vi "Z900_navX_Internal_UpdateDevice.vi"(8 "error in (no error)":errorcluster, 10 "Interface TypeDefs":T1 {"I2CDevRef"."Device Address" format="%.0x"}, 11 "navX Device":T7={"Interface"={"Protocol"=enum."SERIAL", "Update Rate (4Hz-60Hz)"=4, "navX Open TypeDef"=variant}, "Notify Packet"=refnum, "Loop VI Refnum"=refnum, "Ready to Close Occurrence Refnum"=refnum} {"Interface"."Update Rate (4Hz-60Hz)" min=4 max=60 step=1}) -> (0 "error out":errorcluster, 2 "Interface TypeDefs":T1 {"I2CDevRef"."Device Address" format="%.0x"}, 3 "navX Device":T7={"Interface"={"Protocol"=enum."SERIAL", "Update Rate (4Hz-60Hz)"=4, "navX Open TypeDef"=variant}, "Notify Packet"=refnum, "Loop VI Refnum"=refnum, "Ready to Close Occurrence Refnum"=refnum} {"Interface"."Update Rate (4Hz-60Hz)" min=4 max=60 step=1})   [LabVIEW 2015, in "navX Library v2.lvlib"]
doc: "This navX VI handles updating rate and serial protocol for the navX.\nTHIS VI SHOULD NOT BE CALLED BY THE USER!"
uses:
  navX Library v2.lvlib
  TypeDefs/Z900_navX_DeviceTypeDef.ctl
  TypeDefs/Z900_navX_ProtocolTypeDef.ctl
  TypeDefs/Z900_navX_NotifyPacketTypeDef.ctl
  TypeDefs/Z900_navX_ActionTypeDef.ctl
  TypeDefs/Z900_navX_InterfaceTypeDef.ctl
  <vilib>/Rock Robotics/WPI/SerialPort/WPI_SerialPortRef.ctl
  <vilib>/Rock Robotics/WPI/I2C/WPI_I2CDevRef.ctl
  <vilib>/Rock Robotics/SystemInterfaces/i2clib/i2c_bus.ctl
  <vilib>/Rock Robotics/WPI/SPI/WPI_SPIDevRef.ctl
  <vilib>/Rock Robotics/SystemInterfaces/spilib/spi_bus.ctl
  TypeDefs/navX Open TypeDefs/Z900_navX_OpenTypeDef_Serial.ctl
  NI WPI/WPI_SerialPort_USB.ctl
  TypeDefs/Z900_navX_SerialStreamTypeDef.ctl
  TypeDefs/navX Open TypeDefs/Z900_navX_OpenTypeDef_I2C.ctl
  TypeDefs/Z900_navX_DeviceRegisters.ctl
  TypeDefs/navX Open TypeDefs/Z900_navX_OpenTypeDef_SPI.ctl
  Desktop/Library Fix Test/NI WPI/NI WPI Serial USB.lvlib
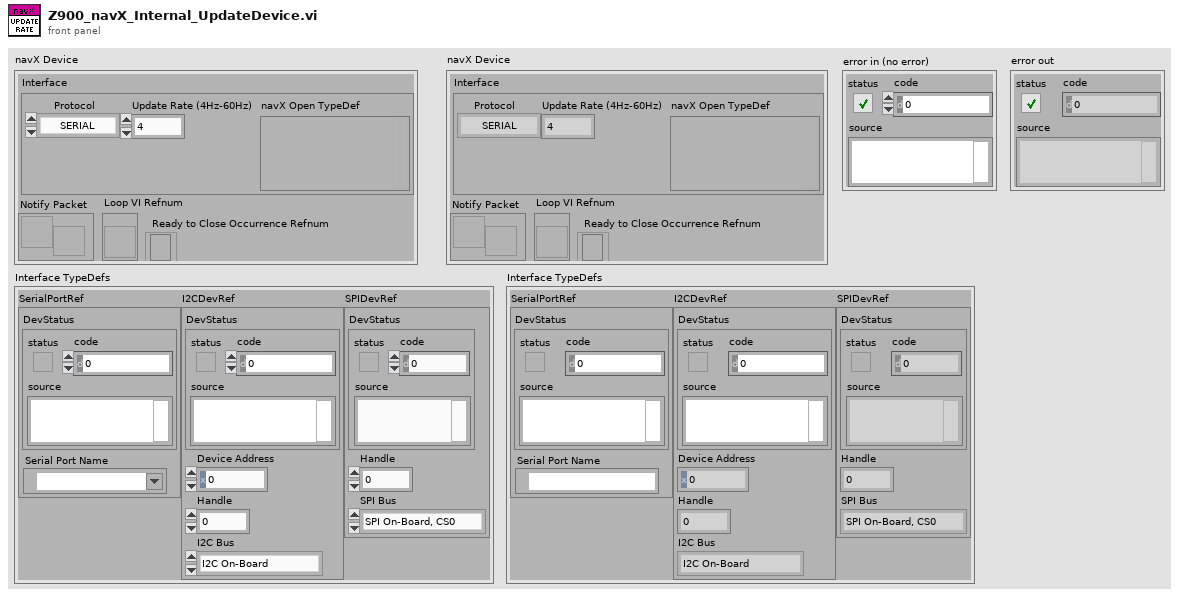
[diagram p1: front panel]
types:
  T1 = typedef "navX Library v2.lvlib/Z900_navX_InterfaceTypeDef.ctl" = cluster{"SerialPortRef":T2, "I2CDevRef":T3, "SPIDevRef":T5}
  T2 = typedef "WPI_SerialPortRef.ctl" = cluster{"DevStatus":errorcluster, "Serial Port Name":refnum<visa-resource-name>}
  T3 = typedef "WPI_I2CDevRef.ctl" = cluster{"DevStatus":errorcluster, "Device Address":u8, "Handle":i32, "I2C Bus":T4}
  T4 = typedef "i2c_bus.ctl" = enum16{"I2C On-Board", "I2C MXP", "Invalid"}
  T5 = typedef "WPI_SPIDevRef.ctl" = cluster{"DevStatus":errorcluster, "Handle":i32, "SPI Bus":T6}
  T6 = typedef "spi_bus.ctl" = enum16{"SPI On-Board, CS0", "SPI On-Board, CS1", "SPI On-Board, CS2", "SPI On-Board, CS3", "SPI MXP", "Invalid"}
  T7 = typedef "navX Library v2.lvlib/Z900_navX_DeviceTypeDef.ctl" = cluster{"Interface":cluster{"Protocol":T8, "Update Rate (4Hz-60Hz)":u8, "navX Open TypeDef":variant}, "Notify Packet":refnum<notifier>, "Loop VI Refnum":refnum<vi>, "Ready to Close Occurrence Refnum":refnum<k4>}
  T8 = typedef "navX Library v2.lvlib/Z900_navX_ProtocolTypeDef.ctl" = enum16{"SERIAL", "I2C", "SPI"}
  T9 = typedef "navX Library v2.lvlib/Z900_navX_OpenTypeDef_Serial.ctl" = cluster{"Serial Port":T10, "Stream Type":T11}
  T10 = typedef "NI WPI Serial USB.lvlib/WPI_SerialPort_USB.ctl" = enum16{"Onboard RS-232", "MXP TTL", "USB"}
  T11 = typedef "navX Library v2.lvlib/Z900_navX_SerialStreamTypeDef.ctl" = enum16{"YRPH", "Quaterinons", "Gyro/Raw", "AHRS", "AHRSAndPositioning"}
  T12 = typedef "navX Library v2.lvlib/Z900_navX_OpenTypeDef_I2C.ctl" = cluster{"I2C Bus":T4}
  T13 = typedef "navX Library v2.lvlib/Z900_navX_OpenTypeDef_SPI.ctl" = cluster{"SPI Bus":T6, "Clock Rate (Hz)":dbl}
  T14 = typedef "navX Library v2.lvlib/Z900_navX_DeviceRegisters.ctl" = u8
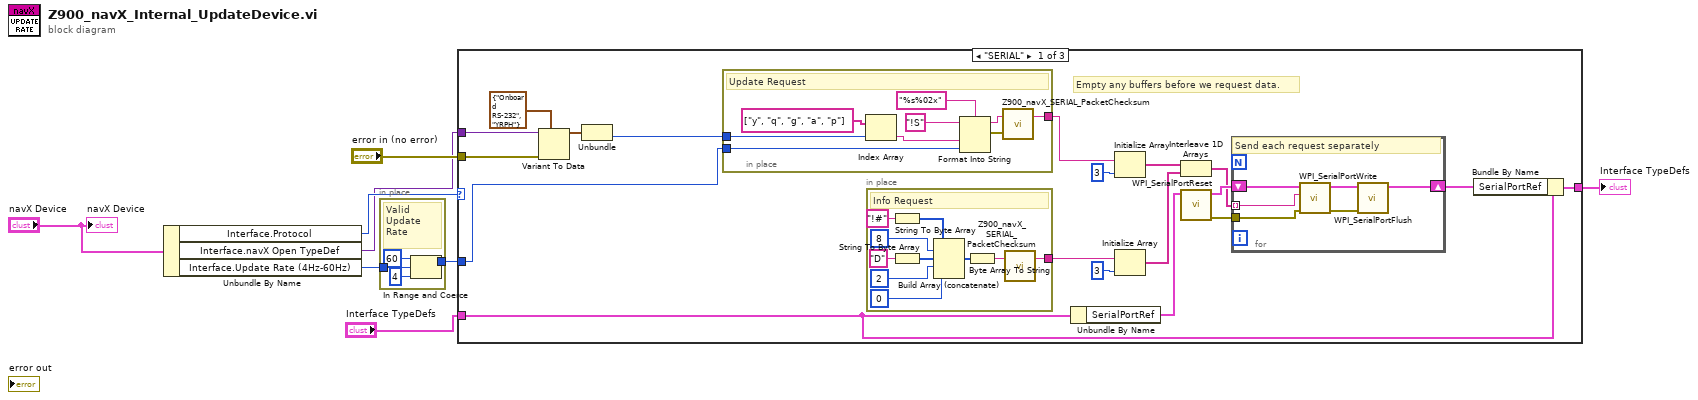
[diagram p0: block diagram]
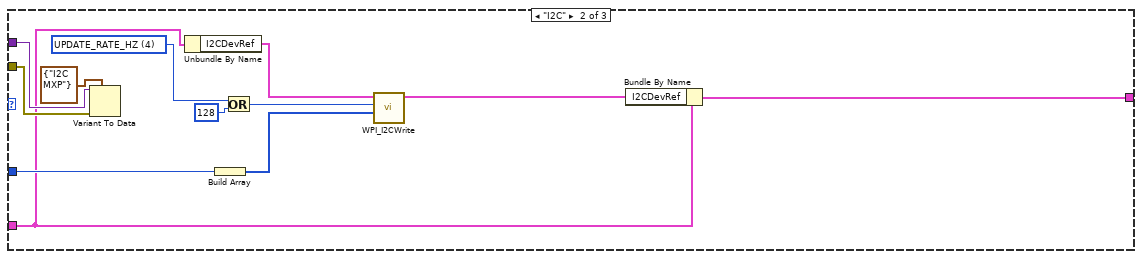
[diagram p2: hidden frame]
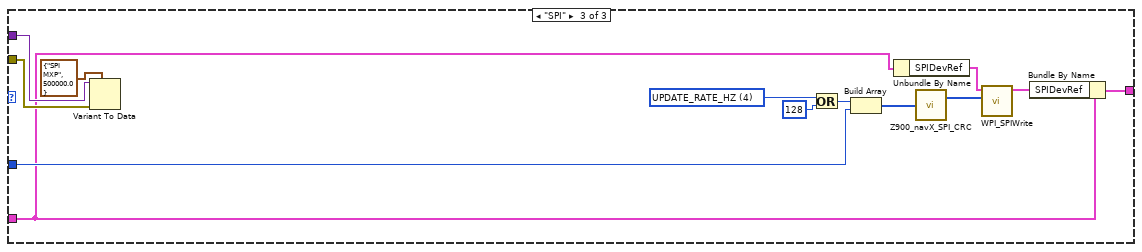
[diagram p3: hidden frame]
diagram:
  n1 = Unbundle By Name("navX Device") -> ("Interface.Protocol"=w7:T8, "Interface.navX Open TypeDef"=w3:variant, "Interface.Update Rate (4Hz-60Hz)"=w2:u8)
  n2 = in-place {
    in-place-border: w2 -> [w12]
    in-place-border: [w9] -> w1
    # "Valid\nUpdate\nRate"
    n3 = In Range and Coerce(upper limit=u8 60, x=w12, lower limit=u8 4) -> (coerced(x)=w9:u8)  [unwired: 1 out]
  }
  n4 = case shown="\"SERIAL\"" w7 {
    tunnel: w3 -> [w31 w68 w81]
    tunnel: "error in (no error)" -> [w29 w66 w79]
    tunnel: "Interface TypeDefs" -> [w26 w59 w71]
    tunnel: w1 -> [w24 w62 w73]
    tunnel: [w25 w57 w69] -> w4
    frame "SERIAL" {
      # "Empty any buffers before we request data."
      n5 = Variant To Data(error in=w29, type=T9 {"Serial Port"=enum."Onboard RS-232", "Stream Type"=enum."YRPH"} ("navX Serial Open"), Variant=w31) -> (data=w28:T9)  [unwired: 1 out]
      n6 = Unbundle(w28) -> ("Stream Type"=w27:T11)  [unwired: 1 out]
      n7 = in-place {
        in-place-border: w27 -> [w45]
        in-place-border: [w38] -> w19
        in-place-border: w24 -> [w39]
        # "Update Request"
        n8 = Index Array(array=string[] ["y", "q", "g", "a", "p"], index=w45) -> (element=w40:string)
        n9 = Format Into String(format string="%s%02x", initial string="!S", w40, w39) -> (resulting string=w43:string, error out=w44:errorcluster)  [unwired: 1 in]
        n10 = call "Z900_navX_SERIAL_PacketChecksum.vi"("error in (no error)"=w44, "Packet"=w43) -> ("Terminated Packet"=w38:string)  [unwired: 1 out]
      }
      n11 = in-place {
        in-place-border: [w47] -> w17
        # "Info Request"
        n12 = String To Byte Array(string="!#" ("initial string")) -> (unsigned byte array=w54:u8[])
        n13 = String To Byte Array(string="D" ("initial string")) -> (unsigned byte array=w52:u8[])
        n14 = Build Array (concatenate)(w54, 8, w52, 2, 0) -> (w49:i32[])
        n15 = Byte Array To String(unsigned byte array=w49) -> (string=w48:string)
        n16 = call "Z900_navX_SERIAL_PacketChecksum.vi"("Packet"=w48) -> ("Terminated Packet"=w47:string)  [unwired: 1 in, 1 out]
      }
      n17 = Unbundle By Name(w26) -> ("SerialPortRef"=w22:T2)
      n18 = Initialize Array(w19, 3 ("dimension size")) -> (w16:string[])
      n19 = Initialize Array(w17, 3 ("dimension size")) -> (w15:string[])
      n20 = Interleave 1D Arrays(w16, w15) -> (w14:string[])
      n21 = call <vilib>:"WPI_SerialPortReset.vi"("SerialPortRef"=w22) -> ("error out"=w20:errorcluster, "SerialPortRef"=w21:T2)  [unwired: 9 in]
      n22 = for {
        tunnel: w20 -> [w34]
        tunnel: w14 -> [w33] mode=indexing
        shift-right: [w32] -> w13
        shift-left: w21 -> [w35]
        # "Send each request separately"
        n23 = call <vilib>:"WPI_SerialPortWrite.vi"("error in (no error)"=w34, "Buffer"=w33, "SerialPortRef"=w35) -> ("error out"=w36:errorcluster, "SerialPortRef"=w37:T2)  [unwired: 6 in, 1 out]
        n24 = call <vilib>:"WPI_SerialPortFlush.vi"("error in (no error)"=w36, "SerialPortRef"=w37) -> ("SerialPortRef"=w32:T2)  [unwired: 8 in, 1 out]
      }
      n25 = Bundle By Name(cluster=w26, "SerialPortRef"=w13) -> (w25:T1)
    }
    frame "I2C" {
      w63 = T14 4 items=["WHOAMI"=0, "HW_REV"=1, "FW_VER_MAJOR"=2, "FW_VER_MINOR"=3, "UPDATE_RATE_HZ"=4, "ACCEL_FSR_G"=5, "GYRO_FSR_DPS"=6, "OP_STATUS"=8, "CAL_STATUS"=9, "SELFTEST_STATUS"=10, "CAPABILITY_FLAGS_L"=11, "CAPABILITY_FLAGS_H"=12, "SENSOR_STATUS"=16, "TIMESTAMP"=18, "YAW"=22, "ROLL"=24, "PITCH"=26, "HEADING"=28, "FUSED_HEADING"=30, "ALTITUDE_I"=32, "ALTITUDE_D"=34, "LINERA_ACC_X"=36, "LINERA_ACC_Y"=38, "LINERA_ACC_Z"=40, "QUAT_W"=42, "QUAT_X"=44, "QUAT_Y"=46, "QUAT_Z"=48, "MPU_TEMP_C"=50, "GYRO_X"=52, "GYRO_Y"=54, "GYRO_Z"=56, "ACC_X"=58, "ACC_Y"=60, "ACC_Z"=62, "MAG_X"=64, "MAG_Y"=66, "MAG_Z"=68, "PRESSURE_I"=70, "PRESSURE_D"=72, "PRESSURE_TEMP"=74, "YAW_OFFSET"=76, "QUAT_OFFSET_W"=78, "QUAT_OFFSET_X"=80, "QUAT_OFFSET_Y"=82, "QUAT_OFFSET_Z"=84, "INTEGRATION_CONTROL"=86, "VELOCITY_X"=88, "VELOCITY_Y"=92, "VELOCITY_Z"=96, "DISPLACMENT_X"=100, "DISPLACMENT_Y"=104, "DISPLACEMENT_Z"=108] ("Device Register")
      n26 = Variant To Data(error in=w66, type=T12 {"I2C Bus"=enum."I2C MXP"} ("navX I2C Open"), Variant=w68) -> ()  [unwired: 2 out]
      n27 = Unbundle By Name(w59) -> ("I2CDevRef"=w60:T3)
      n28 = Build Array(w62) -> (w61:u8[])
      n29 = Or(x=w63, y=u8 128) -> (x .or. y?=w65:T14)
      n30 = call <vilib>:"WPI_I2CWrite.vi"("I2CDataToSend"=w61, "I2CRegister"=w65, "I2CDevRef"=w60) -> ("I2CDevRef"=w58:T3)  [unwired: 7 in, 1 out]
      n31 = Bundle By Name(cluster=w59, "I2CDevRef"=w58) -> (w57:T1)
    }
    frame "SPI" {
      w75 = T14 4 items=["WHOAMI"=0, "HW_REV"=1, "FW_VER_MAJOR"=2, "FW_VER_MINOR"=3, "UPDATE_RATE_HZ"=4, "ACCEL_FSR_G"=5, "GYRO_FSR_DPS"=6, "OP_STATUS"=8, "CAL_STATUS"=9, "SELFTEST_STATUS"=10, "CAPABILITY_FLAGS_L"=11, "CAPABILITY_FLAGS_H"=12, "SENSOR_STATUS"=16, "TIMESTAMP"=18, "YAW"=22, "ROLL"=24, "PITCH"=26, "HEADING"=28, "FUSED_HEADING"=30, "ALTITUDE_I"=32, "ALTITUDE_D"=34, "LINERA_ACC_X"=36, "LINERA_ACC_Y"=38, "LINERA_ACC_Z"=40, "QUAT_W"=42, "QUAT_X"=44, "QUAT_Y"=46, "QUAT_Z"=48, "MPU_TEMP_C"=50, "GYRO_X"=52, "GYRO_Y"=54, "GYRO_Z"=56, "ACC_X"=58, "ACC_Y"=60, "ACC_Z"=62, "MAG_X"=64, "MAG_Y"=66, "MAG_Z"=68, "PRESSURE_I"=70, "PRESSURE_D"=72, "PRESSURE_TEMP"=74, "YAW_OFFSET"=76, "QUAT_OFFSET_W"=78, "QUAT_OFFSET_X"=80, "QUAT_OFFSET_Y"=82, "QUAT_OFFSET_Z"=84, "INTEGRATION_CONTROL"=86, "VELOCITY_X"=88, "VELOCITY_Y"=92, "VELOCITY_Z"=96, "DISPLACMENT_X"=100, "DISPLACMENT_Y"=104, "DISPLACEMENT_Z"=108] ("Device Register")
      n32 = Variant To Data(error in=w79, type=T13 {"SPI Bus"=enum."SPI MXP", "Clock Rate (Hz)"=500000.0} ("navX SPI Open"), Variant=w81) -> ()  [unwired: 2 out]
      n33 = Or(x=w75, y=u8 128) -> (x .or. y?=w76:T14)
      n34 = Build Array(w76, w73) -> (w77:T14[])
      n35 = Unbundle By Name(w71) -> ("SPIDevRef"=w72:T5)
      n36 = call "Z900_navX_SPI_CRC.vi"("Message"=w77) -> ("Message with CRC"=w78:u8[])  [unwired: 1 out]
      n37 = call <vilib>:"WPI_SPIWrite.vi"("Data To Send"=w78, "SPIDevRef"=w72) -> ("SPIDevRef"=w70:T5)  [unwired: 7 in, 2 out]
      n38 = Bundle By Name(cluster=w71, "SPIDevRef"=w70) -> (w69:T1)
    }
  }
  "Interface TypeDefs" <- w4
  "navX Device" <- "navX Device"
